vi "Waveform data to DRAM.vi"(0 "packer out":T1, 1 "Element address input":u32, 2 "Package input valid?":bool, 3 "All points written?":bool) -> (8 "Input ready":bool)   [LabVIEW 2015]
uses:
  <vilib>/rvi/DataTransferAndStorage/Container/Common/niFpgaContainerExecOnDevCompGetState.vi
  <vilib>/rvi/DataTransferAndStorage/Container/Common/niFpgaContainerGetUniqueNameForEmu.vi
  <vilib>/rvi/Memory/Memory_Emulation/niFpgaMemoryEmulationDramWriteAndRequestDataApplyByteEnables.vi
  <vilib>/rvi/Memory/Memory_Emulation/niFpgaMemoryEmulationCacheClearOnFirstRun.vi
  <vilib>/rvi/Memory/Memory_Emulation/nirvimemoryEmulationManagerCache_MakeExclusive.vi
  <vilib>/rvi/Memory/Memory_Emulation/nirvimemoryEmulationManagerCache_GetValue.vi
  <vilib>/rvi/Memory/Memory_Emulation/nirvimemoryEmulationManagerCache_InsertValue.vi
  <vilib>/Utility/error.llb/Clear Errors.vi
  <vilib>/rvi/Memory/Memory_Emulation/nirvimemoryEmulationManagerCache_ReleaseExclusive.vi
  <vilib>/rvi/Memory/Memory_Emulation/nirvimemoryEmulationManagerCache_SetValue.vi
  <vilib>/rvi/DataTransferAndStorage/Container/XNode/niFpgaContainer.xnode
  <vilib>/rvi/Memory/Memory_Emulation/niFpgaMemoryEmulationDramWriteAndRequestDataRefIn.vi
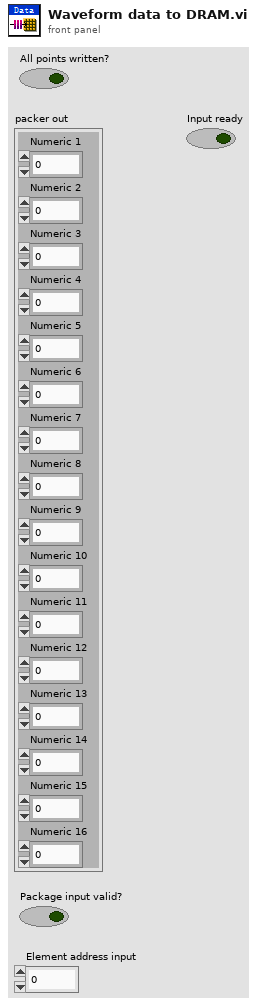
[diagram p1: front panel]
types:
  T1 = cluster{"Numeric 1":u32, "Numeric 2":u32, "Numeric 3":u32, "Numeric 4":u32, "Numeric 5":u32, "Numeric 6":u32, "Numeric 7":u32, "Numeric 8":u32, "Numeric 9":u32, "Numeric 10":u32, "Numeric 11":u32, "Numeric 12":u32, "Numeric 13":u32, "Numeric 14":u32, "Numeric 15":u32, "Numeric 16":u32}
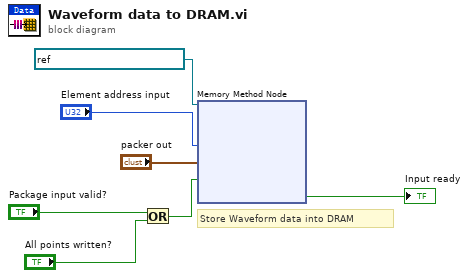
[diagram p0: block diagram]
diagram:
  # "Store Waveform data into DRAM"
  n1 = Or(x="Package input valid?", y="All points written?") -> (x .or. y?=w5:bool)
  n2 = xnode ("Memory Method Node")("地址"="Element address input", "数据"="packer out", "输入有效"=w5, "存储器输入"=refnum<k21> "DRAM for Waveform") -> ("输入就绪"=→"Input ready":bool)  [unwired: 1 out]
